vi "Get Connected System.vi"(8 "error in (no error)":errorcluster, 10 "Connected System":string, 11 "Cobra GUI in":refnum<class "Cobra GUI.lvclass">) -> (0 "error out":errorcluster, 3 "Cobra GUI out":refnum<class "Cobra GUI.lvclass">)   [LabVIEW 2019, in "Cobra GUI.lvlib" / "Cobra GUI.lvclass"]
uses:
  Cobra GUI.lvclass
  <vilib>/regexp/Match Regular Expression.xnode
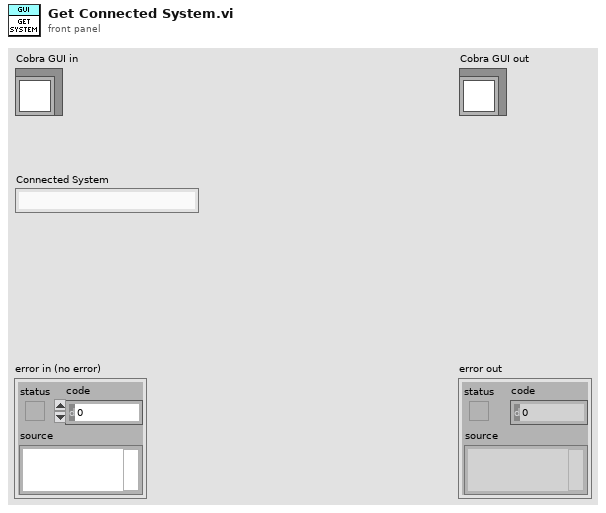
[diagram p1: front panel]
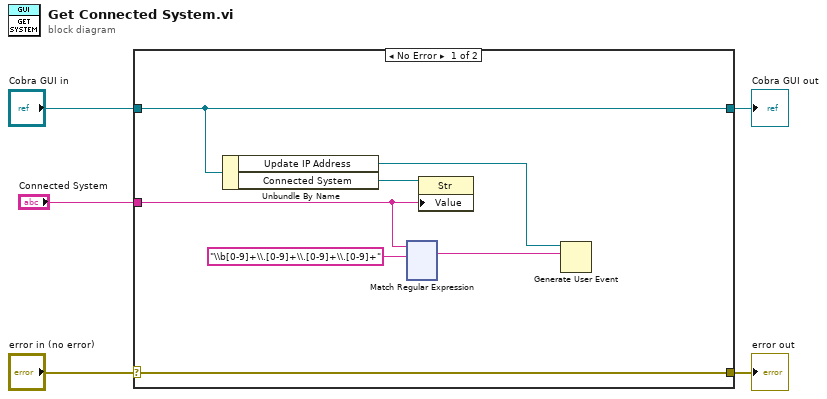
[diagram p0: block diagram]
diagram:
  n1 = case shown="No Error" "error in (no error)" {
    selector: "error in (no error)" -> [w12 w128]
    tunnel: [w12 w128] -> w4
    tunnel: [w10 w127] -> w2
    tunnel: "Cobra GUI in" -> [w10 w127]
    tunnel: "Connected System" -> [w7 _]
    frame No Error {
      n2 = Unbundle By Name(w10) -> ("Update IP Address"=w9:refnum<user-event>, "Connected System"=w11:refnum<vi>)
      n3 = xnode ("Match Regular Expression")("input string"=w7, "regular expression"="\\b[0-9]+\\.[0-9]+\\.[0-9]+\\.[0-9]+") -> ("whole match"=w6:string)  [unwired: 4 in, 4 out]
      n4 = property class="Str"(reference=w11, "Value"=w7) -> ()  [unwired: 1 in, 2 out]
      n5 = Generate User Event(user event=w9, event data cluster=w6) -> ()  [unwired: 2 in, 2 out]
    }
    frame Error {
    }
  }
  "error out" <- w4
  "Cobra GUI out" <- w2
